vi "SPD.Measurments.vi"(5 "Current Progress":refnum<vi>, 6 "Overall Progress":refnum<vi>, 7 "Continue":refnum<vi>, 8 "Error In":errorcluster, 11 "SPD.Stand Ctrl in":T1 {"spdDeviceSession"."hidSPD.Sturtup Values"."HV_bias" format="%#_6p, V"; "spdDeviceSession"."hidSPD.Sturtup Values"."TSet" format="%#_6p, DegC"; "spdDeviceSession"."hidSPD.Controller"."HV_bias" format="%#_6p, V"; "spdDeviceSession"."hidSPD.Controller"."TSet" format="%#_6p, DegC"}) -> (0 "Error Out":errorcluster, 2 "pass":bool, 3 "SPD.Stand Ctrl out":T1 {"spdDeviceSession"."hidSPD.Sturtup Values"."HV_bias" format="%#_6p, V"; "spdDeviceSession"."hidSPD.Sturtup Values"."TSet" format="%#_6p, DegC"; "spdDeviceSession"."hidSPD.Controller"."HV_bias" format="%#_6p, V"; "spdDeviceSession"."hidSPD.Controller"."TSet" format="%#_6p, DegC"})   [LabVIEW 2018]
uses:
  typedefs/SPD.Stand Ctrl.ctl
  Instruments/SPD HID Interface/hidSPDLibForLabView/LibVIs/hidSPD Controls/hidSPD Device Session.ctl
  Instruments/SPD HID Interface/hidSPDLibForLabView/LibVIs/hidSPD Controls/hidSPD Controller.ctl
  Instruments/SPD HID Interface/hidSPDLibForLabView/LibVIs/hidSPD Controls/hidSPD SPD Type.ctl
  Instruments/KC705 DevBoard/typedefs/DevB.Session.ctl
  Instruments/KeySight 53230A/typedefs/FreqC.Session.ctl
  Instruments/KeySight 8164B/KeySight 8164B LAN InstrLib/typedefs/KeySight 8164B control.ctl
  Instruments/LeCroy SDA830/typedefs/LeCroy.Session.ctl
  typedefs/SPD.Events.ctl
  ConfigFile/SPD.Config File ctrl.ctl
  <vilib>/Utility/config.llb/Config Data RefNum.ctl
  typedefs/SPD.Meas Result.ctl
  typedefs/SPD.Queues.ctl
  typedefs/SPD.Stand state.ctl
  Instruments/KeySight 8164B/KeySight 8164B LAN InstrLib.lvlib
  <vilib>/Utility/config.llb/NI_LVConfig.lvlib
  Instruments/SPD HID Interface/hidSPDLibForLabView/hidSPDLibForLabView.lvlib
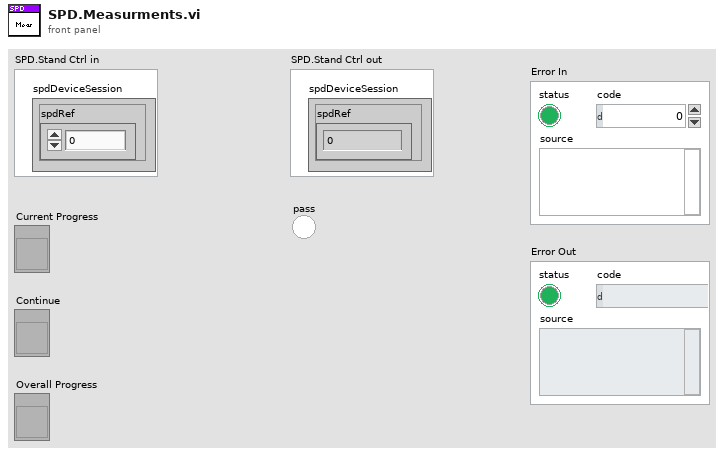
[diagram p1: front panel]
types:
  T1 = typedef "SPD.Stand Ctrl.ctl" = cluster{"spdDeviceSession":T2, "DevBSession":T5, "FreqCSession":T6, "8164BSession":T7, "LeCroySession":T8, "Events":T9, "configFile":T10, "SPD.Result":T12, "SPD.Queues":T13, "Console":refnum<vi>}
  T2 = typedef "hidSPDLibForLabView.lvlib/hidSPD Device Session.ctl" = cluster{"spdRef":u64, "connected":bool, "spdName":string, "hidSPD.Controller":T3, "hidSPD.Sturtup Values":T3, "SPD Type":T4}
  T3 = typedef "hidSPDLibForLabView.lvlib/hidSPD Controller.ctl" = cluster{"TSet":sgl, "HV_bias":sgl, "DDS_stb_code":u16}
  T4 = typedef "hidSPDLibForLabView.lvlib/hidSPD SPD Type.ctl" = enum16{"Free Run", "Gate"}
  T5 = typedef "DevB.Session.ctl" = cluster{"DevBRef":refnum<visa-resource-name>, "connected":bool}
  T6 = typedef "FreqC.Session.ctl" = cluster{"FreqCRef":refnum<visa-resource-name>, "timeout":dbl, "Gate":dbl, "connected":bool}
  T7 = typedef "KeySight 8164B LAN InstrLib.lvlib/KeySight 8164B control.ctl" = cluster{"Connection ID":refnum<k5>, "Connected":bool, "Info":string, "Slots Info":string[]}
  T8 = typedef "LeCroy.Session.ctl" = cluster{"LeCroySession":refnum<visa-resource-name>, "connected":bool}
  T9 = typedef "SPD.Events.ctl" = cluster{"DCRTest":refnum<user-event>, "Stop":refnum<user-event>}
  T10 = typedef "SPD.Config File ctrl.ctl" = cluster{"configFile ref":T11, "configFile path":path, "equipmentFile ref":T11}
  T11 = typedef "NI_LVConfig.lvlib/Config Data RefNum.ctl" = refnum<k1>
  T12 = typedef "SPD.Meas Result.ctl" = cluster{"HV_Bias":dbl[][][], "Stb_code":dbl[], "Temprature":dbl[], "Data":dbl[][][][], "DateTime":string}
  T13 = typedef "SPD.Queues.ctl" = cluster{"state queue":refnum<queue>}
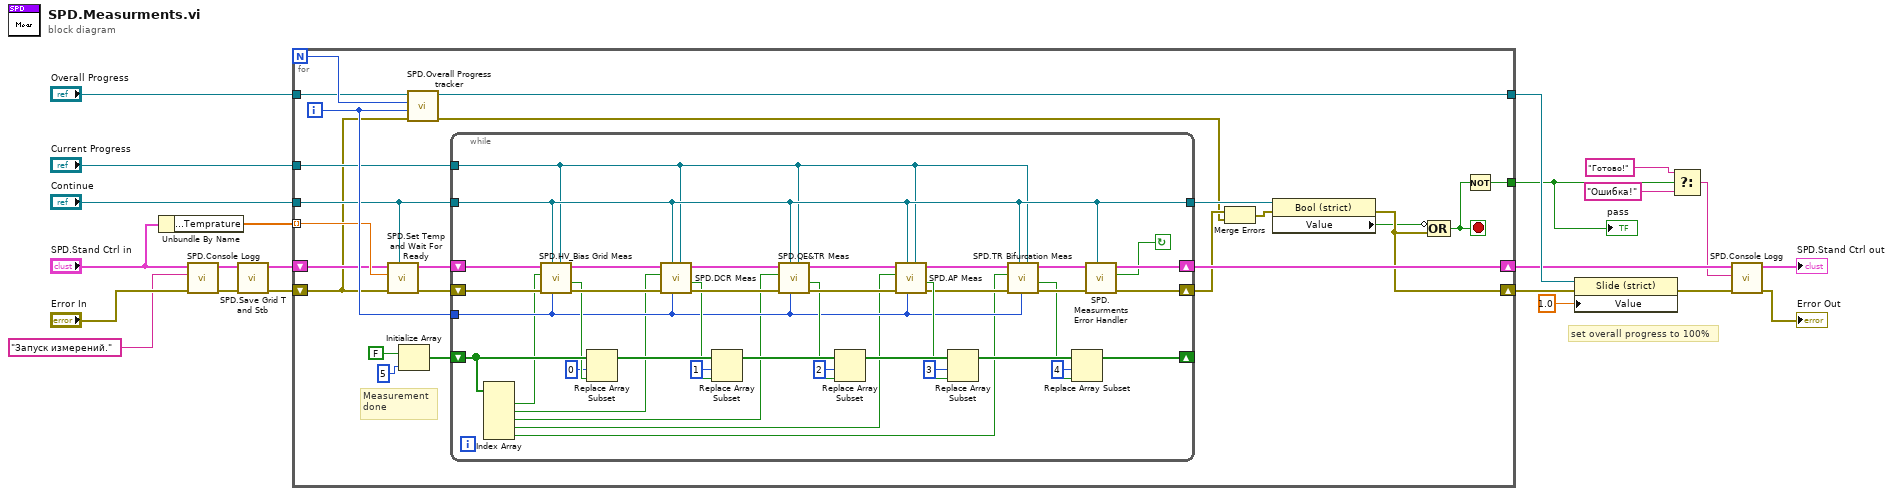
[diagram p0: block diagram]
diagram:
  # "set overall progress to 100%"
  n1 = Unbundle By Name("SPD.Stand Ctrl in") -> ("SPD.Result.Temprature"=w18:dbl[])
  n2 = call "SPD.Console Logg.vi"("Error In"="Error In", "console Log"="Запуск измерений.", "SPD.Stand Ctrl in"="SPD.Stand Ctrl in") -> ("Error Out"=w11:errorcluster, "SPD.Stand Ctrl out"=w12:T1)  [unwired: 7 in]
  n3 = call "SPD.Save Grid T and Stb.vi"("Error In"=w11, "SPD.Stand Ctrl in"=w12) -> ("Error Out"=w21:errorcluster, "SPD.Stand Ctrl out"=w22:T1)  [unwired: 8 in]
  n4 = for {
    N -> [w43]
    shift-right: [w45] -> w6
    shift-left: w22 -> [w38]
    shift-right: [w30] -> w2
    shift-left: w21 -> [w25]
    tunnel: w18 -> [w39] mode=indexing
    tunnel: [w27] -> w7
    tunnel: "Current Progress" -> [w42]
    tunnel: "Continue" -> [w41]
    tunnel: "Overall Progress" -> [w40]
    tunnel: [w26] -> w16
    i -> [w44]
    stop <- w28 stop-if-true
    # "Measurement\ndone"
    n5 = call "SPD.Set Temp and Wait For Ready.vi"("Continue"=w41, "Error In"=w25, "Tset"=w39, "SPD.Stand Ctrl in"=w38) -> ("Error Out"=w36:errorcluster, "SPD.Stand Ctrl out"=w37:T1)  [unwired: 6 in]
    n6 = Initialize Array(FALSE, 5 ("dimension size")) -> (w33:bool[])
    n7 = call "SPD.Overall Progress tracker.vi"("Error In"=w25, "Num of temps"=w44, "Current temprature index"=w43, "Slide in"=w40) -> ("Error Out"=w23:errorcluster, "Slide out"=w26:refnum<vi>)  [unwired: 6 in]
    n8 = while {
      tunnel: w44 -> [w55]
      tunnel: w42 -> [w58]
      tunnel: w41 -> [w59]
      shift-right: [w64] -> w45
      shift-left: w37 -> [w78]
      shift-right: [w63] -> w31
      shift-left: w36 -> [w77]
      shift-right: [w52] -> _
      shift-left: w33 -> [w76]
      tunnel: [w59] -> w32
      stop <- w62 continue-if-true
      n9 = Index Array(array=w76) -> (element #1=w48:bool, element #2=w49:bool, element #3=w50:bool, element #4=w47:bool, element #5=w46:bool)  [unwired: 5 in]
      n10 = call "SPD.HV_Bias Grid Meas.vi"("Progress"=w58, "Temperature index"=w55, "Continue"=w59, "Error In"=w77, "Already done"=w48, "SPD.Stand Ctrl in"=w78) -> ("Error Out"=w83:errorcluster, "done"=w75:bool, "SPD.Stand Ctrl out"=w84:T1)  [unwired: 2 in, 1 out]
      n11 = Replace Array Subset(array=w76, new element=w75, index=0) -> (w73:bool[])
      n12 = call "SPD.DCR Meas.vi"("Progress"=w58, "Temperature index"=w55, "Continue"=w59, "Error In"=w83, "Already done"=w49, "SPD.Stand Ctrl in"=w84) -> ("Error Out"=w81:errorcluster, "pass"=w72:bool, "SPD.Stand Ctrl out"=w82:T1)  [unwired: 2 in, 1 out]
      n13 = Replace Array Subset(array=w73, new element=w72, index=1) -> (w70:bool[])
      n14 = call "SPD.QE&TR Meas.vi"("Progress"=w58, "Temperature index"=w55, "Continue"=w59, "Error In"=w81, "Already done"=w50, "SPD.Stand Ctrl in"=w82) -> ("Error Out"=w79:errorcluster, "pass"=w68:bool, "SPD.Stand Ctrl out"=w80:T1)  [unwired: 2 in, 1 out]
      n15 = Replace Array Subset(array=w70, new element=w68, index=2) -> (w66:bool[])
      n16 = call "SPD.AP Meas.vi"("Progress"=w58, "Temperature index"=w55, "Continue"=w59, "Error In"=w79, "Already done"=w47, "SPD.Stand Ctrl in"=w80) -> ("Error Out"=w60:errorcluster, "pass"=w65:bool, "SPD.Stand Ctrl out"=w61:T1)  [unwired: 2 in, 1 out]
      n17 = Replace Array Subset(array=w66, new element=w65, index=3) -> (w53:bool[])
      n18 = call "SPD.TR Bifurcation Meas.vi"("Progress"=w58, "Temperature index"=w55, "Continue"=w59, "Error In"=w60, "Already done"=w46, "SPD.Stand Ctrl in"=w61) -> ("Error Out"=w56:errorcluster, "pass"=w51:bool, "SPD.Stand Ctrl out"=w57:T1)  [unwired: 2 in, 1 out]
      n19 = Replace Array Subset(array=w53, new element=w51, index=4) -> (w52:bool[])
      n20 = call "SPD.Measurments Error Handler.vi"("Continue"=w59, "Error In"=w56, "SPD.Stand Ctrl in"=w57) -> ("Error Out"=w63:errorcluster, "Re-Measure"=w62:bool, "SPD.Stand Ctrl out"=w64:T1)  [unwired: 6 in]
    }
    n21 = Merge Errors(w31, w23) -> (w24:errorcluster)
    n22 = property class="Bool (strict)"(reference=w32, error in=w24) -> (error out=w30:errorcluster, "Value"=w29:bool)  [unwired: 1 out]
    n23 = Compound Arithmetic op=OR(invert w29, w30) -> (w28:bool)
    n24 = Not(x=w28) -> (.not. x?=w27:bool)
  }
  "pass" <- w7
  n25 = property on="Property Node" class="Slide (strict)"(reference=w16, error in=w2, "Value"=1.0) -> (error out=w1:errorcluster)  [unwired: 1 out]
  n26 = Select(t="Готово!" ("Report"), s=w7, f="Ошибка!") -> (s? t:f=w5:string)
  n27 = call "SPD.Console Logg.vi"("Error In"=w1, "console Log"=w5, "SPD.Stand Ctrl in"=w6) -> ("Error Out"=→"Error Out":errorcluster, "SPD.Stand Ctrl out"=→"SPD.Stand Ctrl out":T1)  [unwired: 7 in]
